vi "LVClass_Camera get CameraSet.vi"(0 "Camera in":refnum<class "Camera.lvclass">, 11 "error in (no error)":errorcluster) -> (4 "Camera out":refnum<class "Camera.lvclass">, 6 "CameraSet.lvclass":refnum<class "CameraSet.lvclass">, 15 "error out":errorcluster)   [LabVIEW 2020, in "Camera.lvclass"]
doc: "Ask camera for array_size captures and retrieve images array (Synchronous mode\n- Blocking).\n\n--------------------------------------------------------------------------------\n\n<B>CameraIn</B> : Camera object.\n\n<B>CameraOut</B> : Camera object.\n\n<B>image_array_size</B> : Captured sequence length (number of cImage).\n\n<B>image_array</B> : Captured sequence as cImage array.\n\n<B>ErrorIn</B> : Error\n\n<B>ErrorOut</B> : Error"
uses:
  Camera.lvclass
  CameraSet/CameraSet.lvclass
  Camera.lvclass/Camera.ctl
  CameraSet/LVClass_CameraSet Write CameraSet.vi
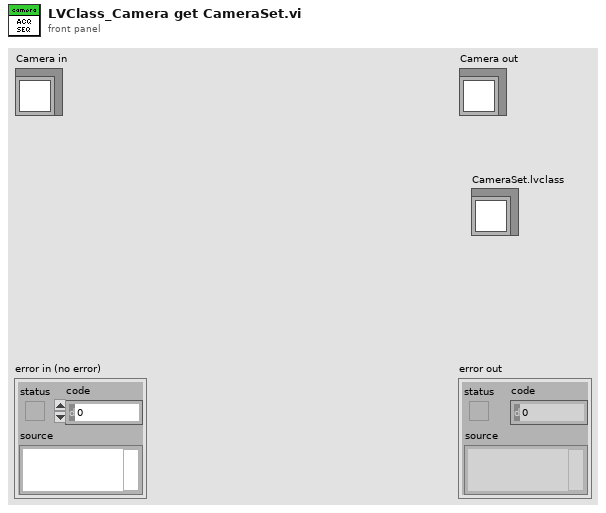
[diagram p1: front panel]
types:
  T1 = typedef "ClassID.ctl" = i64
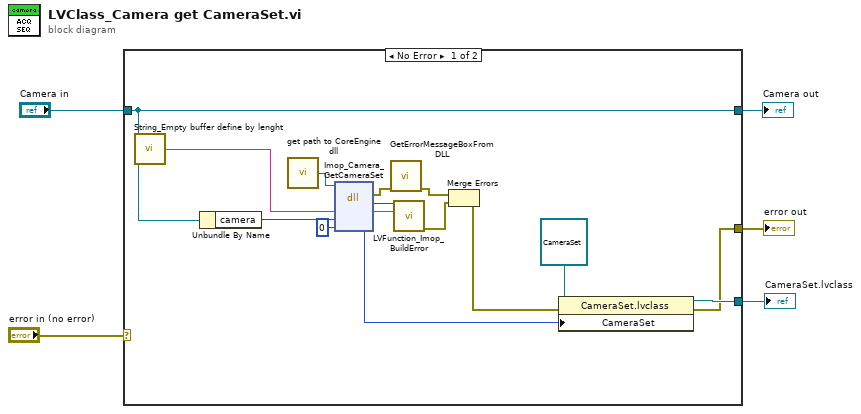
[diagram p0: block diagram]
diagram:
  n1 = case shown="No Error" "error in (no error)" {
    selector: "error in (no error)" -> [_ w22]
    tunnel: [w6 w22] -> w4
    tunnel: [w19 w21] -> w2
    tunnel: "Camera in" -> [w19 w21]
    tunnel: [w8 _] -> w1
    frame No Error {
      n2 = call "String_Empty buffer define by lenght.vi"() -> ("Empty buffer"=w20:string)  [unwired: 1 in]
      n3 = Unbundle By Name(w19) -> ("camera"=w18:T1)
      n4 = call "get path to CoreEngine dll.vi"() -> ("path to wavekit library"=w15:path)  [unwired: 14 in, 1 out]
      n5 = dll-call lib="D:/soft/HASO_v3/SVN_trunk/ImOpCoreEngine4_LV2011/DLLs/c_interface_vc100.dll" fn="Imop_Camera_GetCameraSet"(path in=w15, "message"=w20, "camera"=w18, "CameraSet"=0) -> (error out=w14:errorcluster, "return type"=w16:i32, "message"=w17:string, "CameraSet"=w9:i64)  [unwired: 3 in, 1 out]
      n6 = call "GetErrorMessageBoxFromDLL.vi"("error IN"=w14) -> ("error OUT"=w13:errorcluster)  [unwired: 10 in]
      n7 = call "LVFunction_Imop_BuildError.vi"("code"=w16, "String to Prepend to source (\"\")"=w17) -> ("error out"=w12:errorcluster)  [unwired: 13 in]
      n8 = Merge Errors(w13, w12) -> (w7:errorcluster)
      n9 = property class="CameraSet.lvclass"(reference=refnum<class "CameraSet.lvclass"> refnum ("CameraSet.lvclass"), error in=w7, "CameraSet"=w9) -> (reference out=w8:refnum<class "CameraSet.lvclass">, error out=w6:errorcluster)
    }
    frame Error {
    }
  }
  "error out" <- w4
  "Camera out" <- w2
  "CameraSet.lvclass" <- w1
